vi "Read Signal Generator.lvclass.vi"(11 "Harmonics in":refnum<class "Harmonics.lvclass">) -> (2 "Signal Generator.lvclass":refnum<class "Signal Generator.lvclass">, 3 "Harmonics out":refnum<class "Harmonics.lvclass">)   [LabVIEW 2020, in "Harmonics.lvclass"]
uses:
  Harmonics.lvclass
  Instruments/Signal Generator/Signal Generator.lvclass
  Harmonics.lvclass/Harmonics.ctl
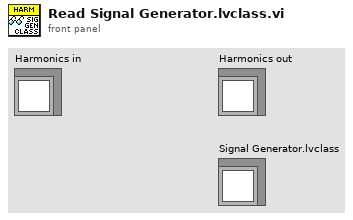
[diagram p1: front panel]
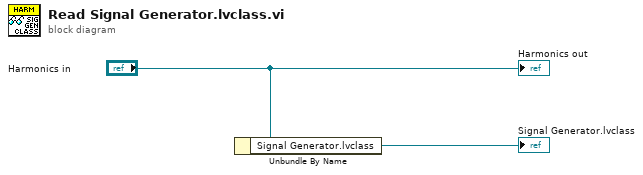
[diagram p0: block diagram]
diagram:
  n1 = Unbundle By Name("Harmonics in") -> ("Signal Generator.lvclass"=→"Signal Generator.lvclass":refnum<class "Signal Generator.lvclass">)
  "Harmonics out" <- "Harmonics in"
